vi "Config UI - Global Stop.vi"(7 "Operation":T1=enum."STOP", 8 "error in (no error)":errorcluster) -> (0 "error out":errorcluster, 3 "Stop?":bool)   [LabVIEW 2011]
uses:
  Controls/Config UI Global Stop - Operations.ctl
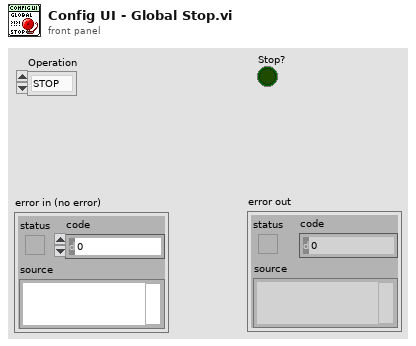
[diagram p1: front panel]
types:
  T1 = typedef "Config UI Global Stop - Operations.ctl" = enum16{"INIT", "STATUS", "STOP"}
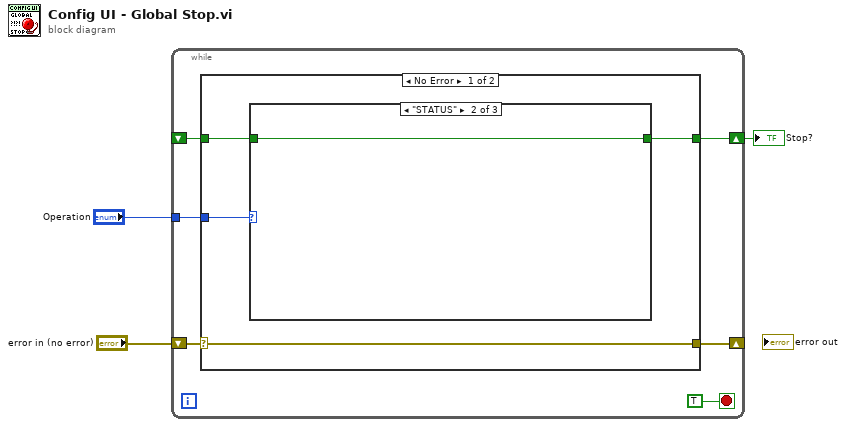
[diagram p0: block diagram]
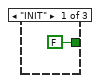
[diagram p2: hidden frame]
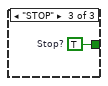
[diagram p3: hidden frame]
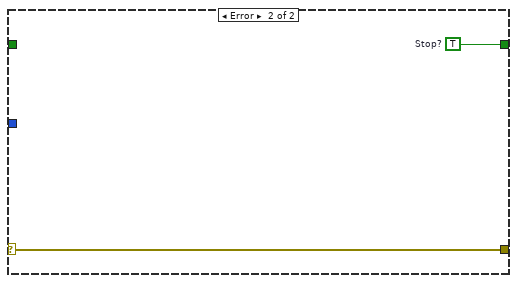
[diagram p4: hidden frame]
diagram:
  n1 = while {
    shift-right: [w8] -> w1
    shift-left: _ -> [w5]
    shift-right: [w7] -> _
    shift-left: "error in (no error)" -> [w9]
    tunnel: "Operation" -> [w4]
    stop <- TRUE stop-if-true
    n2 = case shown="No Error" w9 {
      selector: w9 -> [w11 w17]
      tunnel: [w10 w18] -> w8
      tunnel: [w11 w17] -> w7
      tunnel: w5 -> [w13 _]
      tunnel: w4 -> [w12 _]
      frame No Error {
        n3 = case shown="\"STATUS\"" w12 {
          tunnel: w13 -> [_ w15 _]
          tunnel: [FALSE ("Stop?") w15 w16] -> w10
          frame "INIT" {
          }
          frame "STATUS" {
          }
          frame "STOP" {
            w16 = TRUE  # Stop?
          }
        }
      }
      frame Error {
        w18 = TRUE  # Stop?
      }
    }
  }
  "Stop?" <- w1
